vi "WILT Valve Test.vi"(0 "Water Valves Cluster":T8, 1 "Test Type":T7=enum."Full Valve Control", 2 "Operation Type":T11=enum."Operate As Stand-Alone EXE", 3 "Valve ON Time":dbl=100.0, 5 "Start Buttons Cluster":T9, 7 "Station Test State In":T5, 9 "Station Number":i32, 11 "Error In":errorcluster, 12 "Injection Times":T4, 13 "Day/Night Cycle":T10) -> (4 "Valve Actuation Complete":bool, 6 "Test Station Out":T5, 15 "Error Out":errorcluster)   [LabVIEW 2016]
uses:
  Type Definitions/WILT Water Valve Test Type.ctl
  Type Definitions/WILT Water Valve EXE Operation Type.ctl
  Type Definitions/WILT Water Valve Cluster.ctl
  Type Definitions/WILT Start Button Cluster.ctl
  Type Definitions/WILT Station Test State Cluster.ctl
  Type Definitions/WILT Dryer Test State.ctl
  Type Definitions/WILT Water Injection Control.ctl
  Type Definitions/WILT Day Night Cycle Enum.ctl
  Type Definitions/WILT Agilent Channel Definition.ctl
  Type Definitions/WILT Agilent Data Cluster.ctl
  <vilib>/Utility/error.llb/whitespace.ctl
  Drivers/Agilent 34972/Agilent 34970.lvlib
panel:
  out "Success":bool
  in  "Agilent Data In":T1
  out "Agilent Semaphore":T3[](array[typedef])
  in  "Agilent Switches":T2[](array[typedef])
  in  "Tab Control 2":enum32{"Water Valves", "Page 2"}(tab)
  out "Channel State?":string
  out "Agilent":T3
  in  "Tab Control":enum32{"Valve Setup", "Settings"}(tab)
  in  "Read Data":bool
  in  "Stop All Valves":bool
  in  "Shutdown All":bool
  in  "OK":bool
  in  "Number of ON/OFF Cycles":i32=1
  in  "Delay Before Valve ON":u32
  in  "Current Limit":dbl=1.0
  in  "Current Per Valve":dbl=0.42
  out "Label":string="Water Valve"
  out "Agilent Used":string="3"
  out "Channel Being Used":string="102"
  out "Agilent Data Out":T1
  out "Agilent Array":refnum<visa-resource-name>[](array[refnum])=["AGILENT2", "AGILENT2", "AGILENT2", "AGILENT2", "AGILENT2", "AGILENT2", "AGILENT2", "AGILENT2", "AGILENT2", "AGILENT2", "AGILENT2", "AGILENT2", "AGILENT2", "AGILENT2", "AGILENT2", "AGILENT2", "AGILENT2", "AGILENT2", "AGILENT2", "AGILENT2", "AGILENT3", "AGILENT3", "AGILENT3", "AGILENT3", "AGILENT3", "AGILENT3", "AGILENT3", "AGILENT3", "AGILENT3", "AGILENT3", "AGILENT3", "AGILENT3", "AGILENT5", "AGILENT5", "AGILENT5", "AGILENT5", "AGILENT5", "AGILENT5", "AGILENT5", "AGILENT5", "AGILENT5", "AGILENT5", "AGILENT5", "AGILENT5", "AGILENT5", "AGILENT5", "AGILENT5", "AGILENT5", "AGILENT5", "AGILENT5", "AGILENT5", "AGILENT5", "AGILENT5", "AGILENT5", "AGILENT5", "AGILENT5", "AGILENT5", "AGILENT5", "AGILENT5", "AGILENT5", "AGILENT5", "AGILENT5", "AGILENT5", "AGILENT5", "AGILENT5", "AGILENT5", "AGILENT5", "AGILENT5", "AGILENT7", "AGILENT7", "AGILENT7", "AGILENT7", "AGILENT7", "AGILENT7", "AGILENT7", "AGILENT7", "AGILENT7", "AGILENT7", "AGILENT7", "AGILENT7"]
  out "Agilent Channels":string[](array[string])=["301", "302", "303", "304", "305", "306", "307", "308", "309", "310", "311", "312", "313", "314", "315", "316", "317", "318", "319", "320", "101", "102", "103", "104", "105", "106", "107", "108", "109", "110", "111", "112", "101", "102", "103", "104", "105", "106", "107", "108", "109", "110", "111", "112", "113", "114", "115", "116", "117", "118", "119", "120", "201", "202", "203", "204", "301", "302", "303", "304", "305", "306", "307", "308", "309", "310", "311", "312", "101", "102", "103", "104", "105", "106", "107", "108", "109", "110", "111", "112"]
  out "Start Buttons":string[][](array[string])
  out "Water Valves":string[][](array[string])
  in  "Agilent Channel Assignment":path=path "C:/Work/Agilent Channel Assignment - Wilt.ini"
  out "Message":string
  # "100 ms is good for start switch"
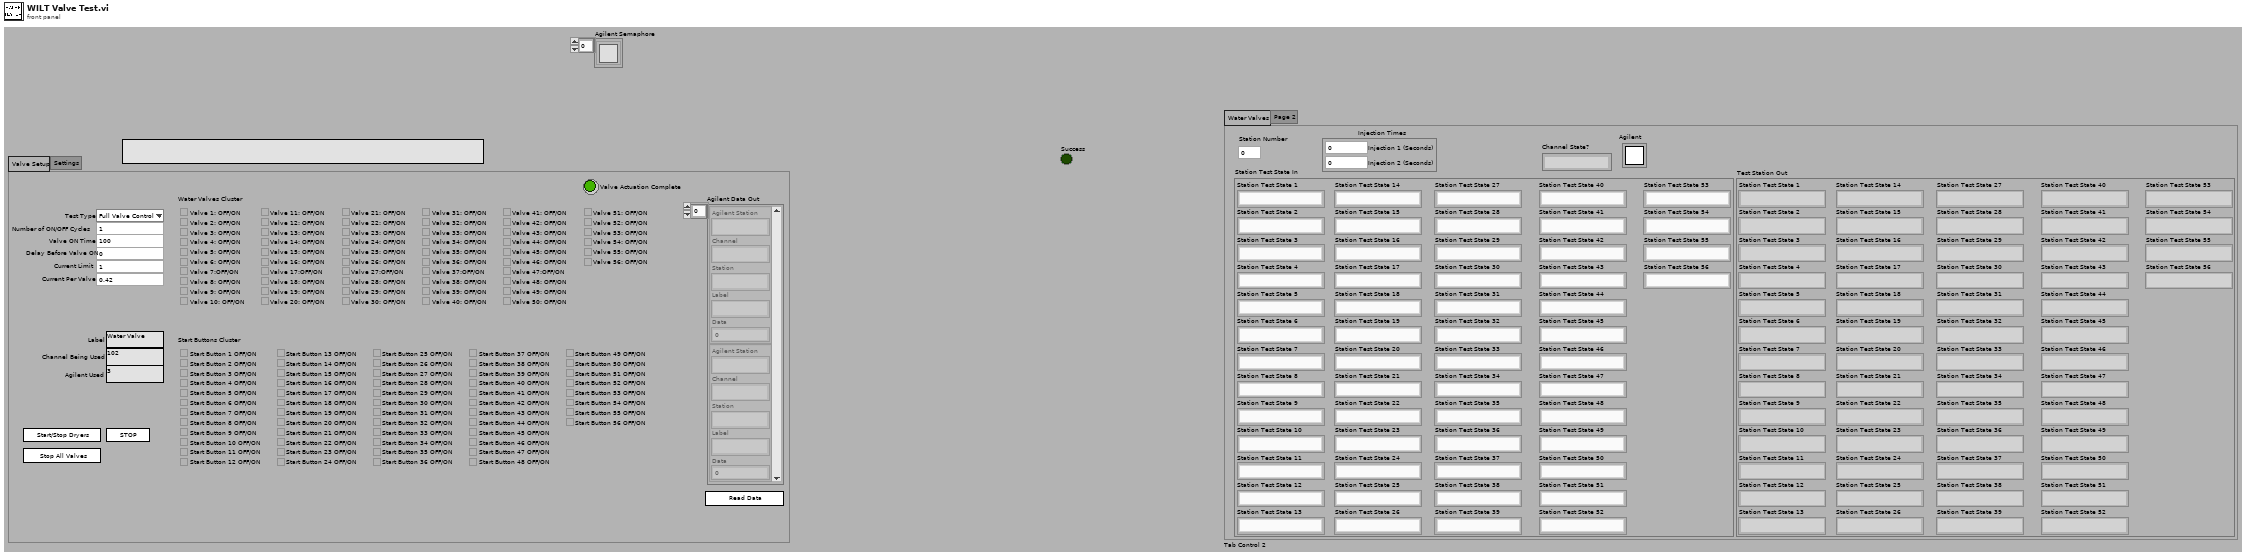
[diagram p1: front panel]
types:
  T1 = typedef "WILT Agilent Data Cluster.ctl" = T2[]
  T2 = typedef "WILT Agilent Channel Definition.ctl" = cluster{"Channel":string, "Station":string, "Label":string, "Agilent Station":string, "Data":dbl}
  T3 = typedef "Semaphore RefNum" = refnum<k1>
  T4 = typedef "WILT Water Injection Control.ctl" = cluster{"Injection 1 (Seconds)":dbl, "Injection 2 (Seconds)":dbl}
  T5 = typedef "WILT Station Test State Cluster.ctl" = cluster{"Station Test State 1":T6, "Station Test State 2":T6, "Station Test State 3":T6, "Station Test State 4":T6, "Station Test State 5":T6, "Station Test State 6":T6, "Station Test State 7":T6, "Station Test State 8":T6, "Station Test State 9":T6, "Station Test State 10":T6, "Station Test State 11":T6, "Station Test State 12":T6, "Station Test State 13":T6, "Station Test State 14":T6, "Station Test State 15":T6, "Station Test State 16":T6, "Station Test State 17":T6, "Station Test State 18":T6, "Station Test State 19":T6, "Station Test State 20":T6, "Station Test State 21":T6, "Station Test State 22":T6, "Station Test State 23":T6, "Station Test State 24":T6, "Station Test State 25":T6, "Station Test State 26":T6, "Station Test State 27":T6, "Station Test State 28":T6, "Station Test State 29":T6, "Station Test State 30":T6, "Station Test State 31":T6, "Station Test State 32":T6, "Station Test State 33":T6, "Station Test State 34":T6, "Station Test State 35":T6, "Station Test State 36":T6, "Station Test State 37":T6, "Station Test State 38":T6, "Station Test State 39":T6, "Station Test State 40":T6, "Station Test State 41":T6, "Station Test State 42":T6, "Station Test State 43":T6, "Station Test State 44":T6, "Station Test State 45":T6, "Station Test State 46":T6, "Station Test State 47":T6, "Station Test State 48":T6, "Station Test State 49":T6, "Station Test State 50":T6, "Station Test State 51":T6, "Station Test State 52":T6, "Station Test State 53":T6, "Station Test State 54":T6, "Station Test State 55":T6, "Station Test State 56":T6}
  T6 = typedef "WILT Dryer Test State.ctl" = enum16{"No Serial Number", "Waiting for Dryer To Start", "Drying Clothes", "Water Injection 1 (On)", "Water Injection 1 Timer", "Water Injection 1 (Off)", "Pause Dryer", "Sending Start Stop CMD", "Pause Dryer 2", "Sending Start Stop CMD 2", "Drying Clothes 2", "Water Injection 2 (On)", "Water Injection 2 Timer", "Water Injection 2 (Off)", "Drying Clothes 3", "Cooling Down", "Sending Start Stop CMD 3", "Increment Cycle"}
  T7 = typedef "WILT Water Valve Test Type.ctl" = enum16{"Cycle Valve Control", "Full Valve Control"}
  T8 = typedef "WILT Water Valve Cluster.ctl" = cluster{"Valve 1":bool, "Valve 2":bool, "Valve 3":bool, "Valve 4":bool, "Valve 5":bool, "Valve 6":bool, "Valve 7":bool, "Valve 8":bool, "Valve 9":bool, "Valve 10":bool, "Valve 11":bool, "Valve 12":bool, "Valve 13":bool, "Valve 14":bool, "Valve 15":bool, "Valve 16":bool, "Valve 17":bool, "Valve 18":bool, "Valve 19":bool, "Valve 20":bool, "Valve 21":bool, "Valve 22":bool, "Valve 23":bool, "Valve 24":bool, "Valve 25":bool, "Valve 26":bool, "Valve 27":bool, "Valve 28":bool, "Valve 29":bool, "Valve 30":bool, "Valve 31":bool, "Valve 32":bool, "Valve 33":bool, "Valve 34":bool, "Valve 35":bool, "Valve 36":bool, "Valve 37":bool, "Valve 38":bool, "Valve 39":bool, "Valve 40":bool, "Valve 41":bool, "Valve 42":bool, "Valve 43":bool, "Valve 44":bool, "Valve 45":bool, "Valve 46":bool, "Valve 47":bool, "Valve 48":bool, "Valve 49":bool, "Valve 50":bool, "Valve 51":bool, "Valve 52":bool, "Valve 53":bool, "Valve 54":bool, "Valve 55":bool, "Valve 56":bool}
  T9 = typedef "WILT Start Button Cluster.ctl" = cluster{"Start Button 21":bool, "Start Button 22":bool, "Start Button 23":bool, "Start Button 24":bool, "Start Button 25":bool, "Start Button 26":bool, "Start Button 27":bool, "Start Button 28":bool, "Start Button 29":bool, "Start Button 30":bool, "Start Button 31":bool, "Start Button 32":bool, "Start Button 33":bool, "Start Button 34":bool, "Start Button 35":bool, "Start Button 36":bool, "Start Button 37":bool, "Start Button 38":bool, "Start Button 39":bool, "Start Button 40":bool, "Start Button 41":bool, "Start Button 42":bool, "Start Button 43":bool, "Start Button 44":bool, "Start Button 12":bool, "Start Button 11":bool, "Start Button 10":bool, "Start Button 9":bool, "Start Button 8":bool, "Start Button 7":bool, "Start Button 6":bool, "Start Button 5":bool, "Start Button 4":bool, "Start Button 3":bool, "Start Button 2":bool, "Start Button 1":bool, "Start Button 20":bool, "Start Button 19":bool, "Start Button 18":bool, "Start Button 17":bool, "Start Button 16":bool, "Start Button 15":bool, "Start Button 14":bool, "Start Button 13":bool, "Start Button 45":bool, "Start Button 46":bool, "Start Button 47":bool, "Start Button 48":bool, "Start Button 49":bool, "Start Button 50":bool, "Start Button 51":bool, "Start Button 52":bool, "Start Button 53":bool, "Start Button 54":bool, "Start Button 55":bool, "Start Button 56":bool}
  T10 = typedef "WILT Day Night Cycle Enum.ctl" = enum16{"Day Cycle", "Night Cycle", "Day Cycle (No Water)"}
  T11 = typedef "WILT Water Valve EXE Operation Type.ctl" = enum16{"Operate As SubVI", "Operate As Stand-Alone EXE", "Shutdown All Dryers"}
  T12 = enum32{"invalid app kind", "Development System", "Run Time System", "Student Edition", "Embedded LabVIEW", "Evaluation", "Custom"}
  T13 = enum32{"Invalid", "Standard", "Closed", "Hidden", "Minimized", "Maximized"}
  T14 = cluster{"Core":cluster{"Current VI Reference":refnum<vi>, "Close Panel on Exit?":bool}, "Valve Array":bool[], "Water Valve Only":bool[], "Agilent":refnum<visa-resource-name>, "Channel":string, "Agilent Switches":T2[], "Agilent Array":refnum<visa-resource-name>[], "Agilent Channel Array":string[], "Start Buttons":string[][], "Water Valves":string[][], "Valve Act Complete":bool, "Water Valves Cluster":T8, "Start Buttons Cluster":T9, "Station Test State In":T5, "Agilent Data In":T1}
  T15 = cluster{"Current VI Reference":refnum<vi>, "Close Panel on Exit?":bool}
  T16 = typedef "whitespace.ctl" = u16
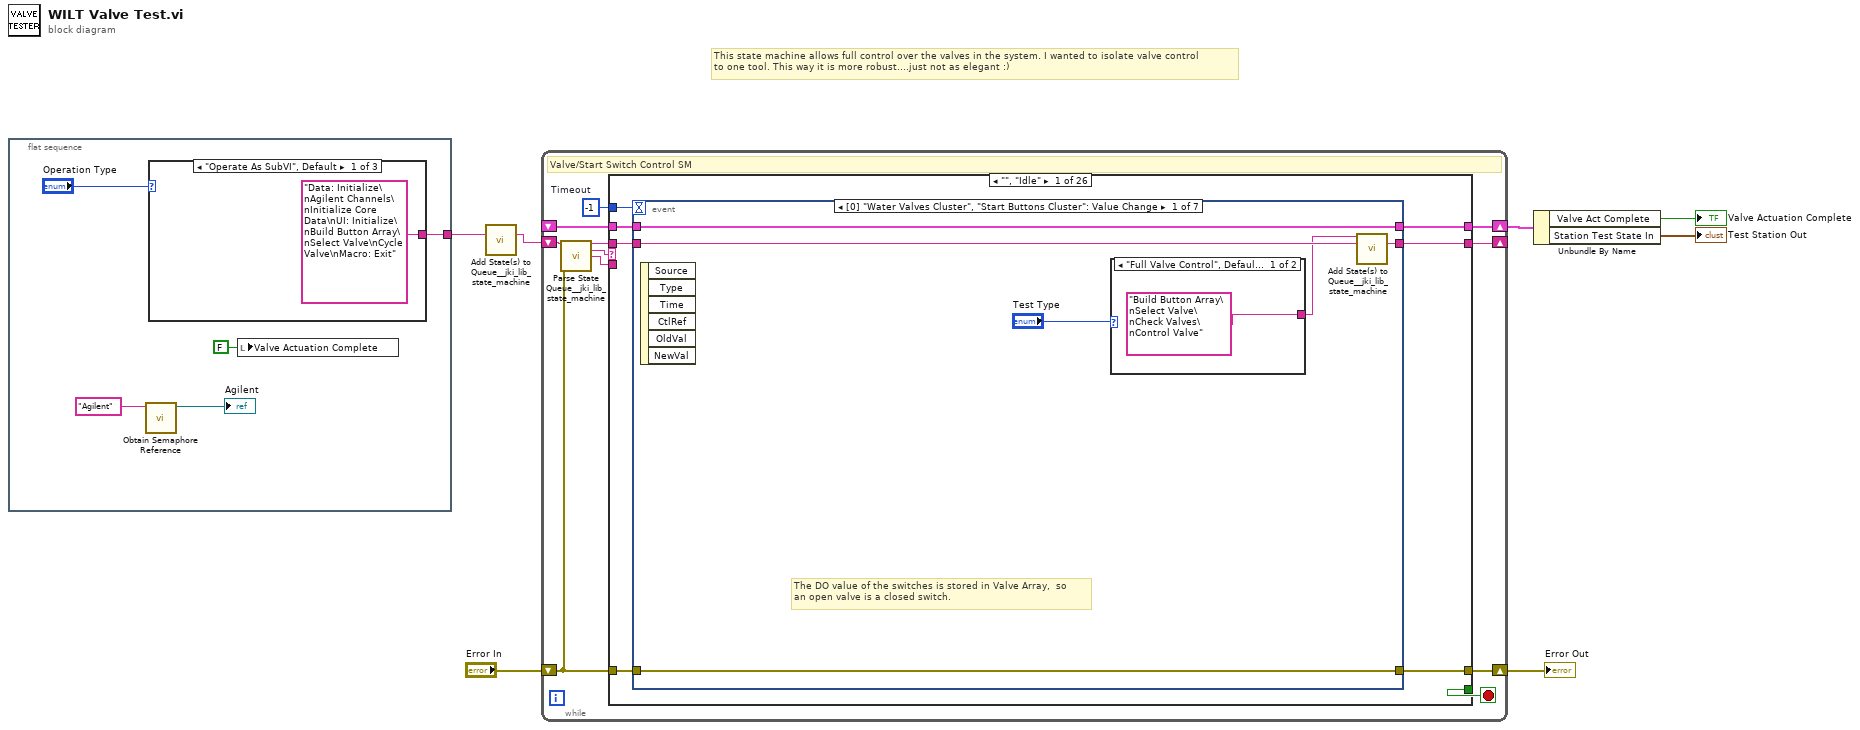
[diagram p0: block diagram]
diagram:
  # "This state machine allows full control over the valves in the system. I wanted to isolate valve control\nto one tool. This way it is more robust....just not as elegant :)"
  n1 = flat-sequence {
    tunnel: [w12] -> w6
    frame #0 {
      n2 = call <vilib>:"Obtain Semaphore Reference.vi"("name (unnamed)"="Agilent") -> ("semaphore"=→"Agilent":T3)  [unwired: 4 in, 2 out]
      n3 = case shown="\"Operate As SubVI\", Default" "Operation Type" {
        tunnel: ["Data: Initialize\nAgilent Channels\nInitialize Core Data\nUI: Initialize\nBuild Button Array\nSelect Valve\nCycle Valve\nMacro: Exit" ("State(s) in Front (\"\")") "Macro: Initialize" "Data: Initialize\nAgilent Channels\nInitialize Core Data\nUI: Initialize\nBuild Button Array\nSelect Valve\nShutdown All\nMacro: Exit" ("State(s) in Front (\"\")")] -> w12
        frame "Operate As SubVI", Default {
        }
        frame "Operate As Stand-Alone EXE" {
        }
        frame "Shutdown All Dryers" {
        }
      }
      n4 = local write "Valve Actuation Complete"(FALSE ("Valve Actuation Complete")) -> ()
    }
  }
  n5 = call <vilib>:"Add State(s) to Queue__jki_lib_state_machine.vi"("State(s) in (\"\")"=w6) -> ("States Out"=w7:string)  [unwired: 14 in]
  n6 = while "Valve/Start Switch Control SM" {
    shift-right: [w19] -> w3
    shift-left: _ -> [w18]
    shift-right: [w22] -> w5
    shift-left: "Error In" -> [w16]
    shift-right: [w21] -> _
    shift-left: w7 -> [w23]
    stop <- w20 stop-if-true
    w17 = -1  # Timeout
    # "Valve/Start Switch Control SM"
    n7 = call <vilib>:"Parse State Queue__jki_lib_state_machine.vi"("State Queue"=w23, "Error In (no error)"=w16) -> ("Remaining States"=w25:string, "Current State"=w26:string, "Arguments"=w24:string)  [unwired: 11 in]
    n8 = case shown="\"\", \"Idle\"" w26 {
      selector: w26 -> [_ _ w77 _ _ _ _ _ _ _ _ _ _ _ _ _ _ _ _ _ _ _ _ _ _ _]
      tunnel: w25 -> [w33 w76 w81 w99 w105 w110 w114 w133 w143 w155 w161 w165 w176 w1545 w1556 w1582 w1587 w1597 w1601 w1617 w1634 w1655 w1706 w1717 w1740 w1753]
      tunnel: w24 -> [_ _ _ _ _ _ _ _ _ _ _ _ _ w1540 w1550 _ _ _ _ _ _ _ _ _ _ _]
      tunnel: w18 -> [w31 w73 w79 w90 w102 w108 w111 _ w141 w147 w156 w162 w168 w1543 w1552 w1579 w1584 w1594 w1598 w1612 w1631 w1646 w1704 w1715 w1735 w1749]
      tunnel: [w30 w74 w83 w96 errorcluster {"status"=FALSE, "code"=0, "source"=""} ("error out") w107 w112 w130 w136 w150 w157 w163 w174 w1541 w1553 w1580 w1585 w1595 w1599 w1615 w1632 w1647 w1703 w1714 w1736 w1751] -> w22
      tunnel: w16 -> [w29 w74 w82 w96 w101 w107 w112 w130 w137 w152 w158 w163 w174 w1542 w1554 w1580 w1585 w1595 w1599 w1615 w1632 w1650 w1702 w1714 w1737 w1751]
      tunnel: [w32 w75 w80 w98 w104 w109 w113 w132 w142 w154 w160 w164 w175 w1544 w1555 w1581 w1586 w1596 w1600 w1616 w1633 w1654 w1705 w1716 w1739 w1752] -> w21
      tunnel: [_ _ _ _ _ TRUE _ _ _ _ _ _ _ _ _ _ _ _ _ _ _ _ _ _ _ _] -> w20
      tunnel: [w28 w73 w79 w97 w102 w108 w111 w131 w140 w146 w156 w162 w172 w1543 w1552 w1579 w1584 w1594 w1598 w1611 w1631 w1645 w1704 w1715 w1735 w1749] -> w19
      tunnel: w17 -> [w27 _ _ _ _ _ _ _ _ _ _ _ _ _ _ _ _ _ _ _ _ _ _ _ _ _]
      frame "", "Idle" {
        n9 = event shown="[0] \"Water Valves Cluster\", \"Start Buttons Cluster\": Value Change" {
          selector: _ -> [_ _ _ _ _ _ _]
          dyn-events: _ -> [_ _ _ _ _ _ _]
          timeout: w27 -> [_ _ _ _ _ _ _]
          tunnel: w33 -> [w39 w46 w51 w54 w58 w63 w72]
          tunnel: [w38 w45 w50 w53 w59 w64 w71] -> w32
          tunnel: w31 -> [w34 w43 w48 w55 w57 w65 w69]
          tunnel: [w37 w44 w49 w56 w61 w66 w70] -> w30
          tunnel: w29 -> [w37 w44 w49 w56 w61 w66 w70]
          tunnel: [w34 w43 w48 w55 w57 w65 w69] -> w28
          event Value Change {
            # "The DO value of the switches is stored in Valve Array,  so\nan open valve is a closed switch."
            n10 = event-data() -> ()  [unwired: 1 in, 6 out]
            n11 = case shown="\"Full Valve Control\", Default" "Test Type" {
              tunnel: ["Build Button Array\nSelect Valve\nCheck Valves\nControl Valve" ("State(s) in Front (\"\")") "Build Button Array\nSelect Valve\nCheck Valves\nCycle Valve" ("State(s) in Front (\"\")")] -> w36
              frame "Full Valve Control", Default {
              }
              frame "Cycle Valve Control" {
              }
            }
            n12 = call <vilib>:"Add State(s) to Queue__jki_lib_state_machine.vi"("State(s) in Front (\"\")"=w36, "State(s) in (\"\")"=w39) -> ("States Out"=w38:string)  [unwired: 13 in]
          }
          event Timeout {
            n13 = event-data() -> ()  [unwired: 1 in, 3 out]
            n14 = local write "Valve Actuation Complete"(FALSE ("Valve Actuation Complete")) -> ()
            n15 = call <vilib>:"Add State(s) to Queue__jki_lib_state_machine.vi"("State(s) in (\"\")"=w46) -> ("States Out"=w45:string)  [unwired: 14 in]
          }
          event "OK": Value Change {
            n16 = event-data() -> ()  [unwired: 1 in, 1 out]
            n17 = call <vilib>:"Add State(s) to Queue__jki_lib_state_machine.vi"("State(s) in Front (\"\")"="Macro: Exit", "State(s) in (\"\")"=w51) -> ("States Out"=w50:string)  [unwired: 13 in]
          }
          event "Shutdown All": Value Change {
            n18 = event-data() -> ()  [unwired: 1 in, 6 out]
            n19 = call <vilib>:"Add State(s) to Queue__jki_lib_state_machine.vi"("State(s) in Front (\"\")"="Stop All Valves\nShutdown All" ("State(s) in Front (\"\")"), "State(s) in (\"\")"=w54) -> ("States Out"=w53:string)  [unwired: 13 in]
          }
          event "Stop All Valves": Value Change {
            n20 = event-data() -> ()  [unwired: 1 in, 6 out]
            n21 = call <vilib>:"Add State(s) to Queue__jki_lib_state_machine.vi"("State(s) in Front (\"\")"="Stop All Valves" ("State(s) in Front (\"\")"), "State(s) in (\"\")"=w58) -> ("States Out"=w59:string)  [unwired: 13 in]
          }
          event "Read Data": Value Change {
            n22 = event-data() -> ()  [unwired: 1 in, 6 out]
            n23 = call <vilib>:"Add State(s) to Queue__jki_lib_state_machine.vi"("State(s) in Front (\"\")"="Read Agilents" ("name (unnamed)"), "State(s) in (\"\")"=w63) -> ("States Out"=w64:string)  [unwired: 13 in]
          }
          event Panel Close? {
            # "Discard the event because we'll close the front panel ourselves in Macro: Exit"
            # "Close Panel button (pressed) Event\n(this executes Macro: Exit to terminate the VI)"
            n24 = event-data() -> ()  [unwired: 1 in, 1 out]
            n25 = event-data("Discard?"=TRUE) -> ()  [unwired: 1 in, 1 out]
            n26 = call <vilib>:"Add State(s) to Queue__jki_lib_state_machine.vi"("State(s) in Front (\"\")"="Macro: Exit", "State(s) in (\"\")"=w72) -> ("States Out"=w71:string)  [unwired: 13 in]
          }
        }
      }
      frame "---------- Core ----------" {
        # "Do not put any code in this frame.\n(it is a separator no-op)"
        n27 = call <vilib>:"Add State(s) to Queue__jki_lib_state_machine.vi"("State(s) in (\"\")"=w76) -> ("States Out"=w75:string)  [unwired: 14 in]
      }
      frame Default {
        w86 = 42 items=["No error", "Argument error", "Memory is full", "Out of zone", "End of file", "File already open", "Generic file I/O error", "File not found", "File permission error", "Disk is full", "Duplicate path", "Too many files open", "System feature not enabled", "Resource file not found", "Cannot add resource", "Resource not found", "Image not found", "Image memory error", "Pen does not exist", "Config type invalid", "Config token not found", "Config parse error", "Config memory error", "Bad external code format", "Bad external code offset", "External code not present", "Null window", "Destroy window error", "Null menu", "Print aborted", "Bad print record", "Print driver error", "Windows error during printing", "Memory error during printing", "Print dialog error", "Generic print error", "Invalid device refnum", "Device not found", "Device parameter error", "Device unit error", "Cannot open device", "Device call aborted", "Generic error", "Cancelled by user", "Object ID too low", "Object ID too high", "Object not in heap", "Unknown heap", "Unknown object (invalid DefProc)", "Unknown object (DefProc not in table)", "Message out of range", "Invalid (null) method", "Unknown message", "Manager call not supported", "Bad address", "Network operation in progress", "Network operation timed out", "Connection is busy", "Network attribute not supported", "Network error", "Address in use", "System out of memory", "Connection aborted", "Connection refused", "Not connected", "Already connected", "Connection closed", "Initialization error (interapplication manager)", "Bad occurrence", "Wait on unbound occurrence handler", "Occurrence queue overflow", "Datalog type conflict", "Unused", "Unrecognized type (interapplication manager)", "Memory corrupt", "Failed to make temporary DLL", "Old CIN version", "Drag socket not found", "Failed to load drop-object", "Failed to register OLE object", "Failed to release OLE object", "Format specifier type mismatch", "Unknown format specifier", "Too few format specifiers", "Too many format specifiers", "Scan failed", "Newer CIN version", "Error converting to variant", "Runtime menu error", "Password tampered", "Variant attribute not found", "Incompatible variant data type", "Event data is not available", "Event Store is not present", "Occurrence is not found", "Event Queue is not created", "Event info is not available", "Refnum passed is NULL", "Error retrieving Class GUID", "Error retrieving CoClass GUID", "Error retrieving TypeLib GUID.", "Bad built application magic bytes.", "Specific driver is different from the specific driver associated with the Logical Name.", "There is no session opened to the class driver.", "Max Error", "MAX - Error with config objects", "MAX - Error loading configuration", "MAX - Group not supported"]
        # "Current State"
        # "Do not delete, rename, or modify this frame.\n(this is used to capture unhandled states and typos)"
        # "Handle mistyped state name (developer tool)"
        n28 = Format Into String(format string="Software Exception: Unhandled State \"%s\"." ("message"), error in=w82, w77) -> (resulting string=w85:string, error out=w84:errorcluster)  [unwired: 1 in]
        n29 = call <vilib>:"Error Cluster From Error Code.vi"("show call chain? (False)"=TRUE, "error in (no error)"=w84, "error message (\"\")"=w85, "error code (0)"=w86) -> ("error out"=w83:errorcluster)  [unwired: 5 in]
        n30 = call <vilib>:"Add State(s) to Queue__jki_lib_state_machine.vi"("State(s) in (\"\")"=w81) -> ("States Out"=w80:string)  [unwired: 14 in]
      }
      frame "Initialize Core Data" {
        # "Do not delete, rename, or modify this frame.\n(this is used to determine panel behavior on exit)"
        # "originally closed?"
        # "exe?"
        # "If panel starts closed or is an EXE, then close it when we exit"
        n31 = property class="VI"() -> ("Front Panel.Open"=w95:bool)  [unwired: 2 in, 2 out]
        n32 = property class="App"() -> ("App.Kind"=w94:T12)  [unwired: 2 in, 2 out]
        n33 = control-ref of="Current VI Reference"() -> (w88:refnum<vi>)
        n34 = Not(x=w95) -> (.not. x?=w92:bool)
        n35 = Equal?(x=w94, y=T12."Run Time System" ("Application:Kind")) -> (x = y?=w91:bool)
        n36 = Or(x=w92, y=w91) -> (x .or. y?=w89:bool)
        n37 = Bundle By Name(cluster=w90, "Core.Current VI Reference"=w88, "Core.Close Panel on Exit?"=w89) -> (w97:T14)
        n38 = call <vilib>:"Add State(s) to Queue__jki_lib_state_machine.vi"("State(s) in (\"\")"=w99) -> ("States Out"=w98:string)  [unwired: 14 in]
      }
      frame "Error Handler" {
        # "Unhandled Error -- Display it"
        # "Handle any errors here.\nYou can also output any states to clean-up after errors occur"
        # "Clear error"
        n39 = call <vilib>:"General Error Handler.vi"("error in (no error)"=w101) -> ()  [unwired: 10 in, 5 out]
        n40 = call <vilib>:"Add State(s) to Queue__jki_lib_state_machine.vi"("State(s) in Front (\"\")"="/* Post Error States", "State(s) in (\"\")"=w105) -> ("States Out"=w104:string)  [unwired: 13 in]
      }
      frame "Exit" {
        # "Do not put any code in this frame.\n(No errors that occur here will be handled.)"
        n41 = call <vilib>:"Add State(s) to Queue__jki_lib_state_machine.vi"("State(s) in (\"\")"=w110) -> ("States Out"=w109:string)  [unwired: 14 in]
      }
      frame "---------- Data ----------" {
        # "Do not put any code in this frame.\n(It is a separator no-op. You can make a copy of this frame to create a new Data frame)"
        n42 = call <vilib>:"Add State(s) to Queue__jki_lib_state_machine.vi"("State(s) in (\"\")"=w114) -> ("States Out"=w113:string)  [unwired: 14 in]
      }
      frame "Data: Initialize" {
        w121 = bool[] [FALSE, FALSE, FALSE, FALSE, FALSE, FALSE, FALSE, FALSE, FALSE, FALSE]  # Water Valve Only
        w126 = "1"  # Channel
        w127 = refnum<visa-resource-name> "AGILENT1"  # Agilent
        w128 = bool[] [FALSE, FALSE, FALSE, FALSE, FALSE, FALSE, FALSE, FALSE, FALSE, FALSE]  # Valve Array
        w129 = T15 {"Current VI Reference"=refnum, "Close Panel on Exit?"=FALSE}  # Core
        n43 = Bundle("Core"=w129, "Valve Array"=w128, "Water Valve Only"=w121, "Agilent"=w127, "Channel"=w126, "Agilent Switches"="Agilent Switches", "Agilent Array"=refnum<visa-resource-name>[] [], "Agilent Channel Array"=string[] [], "Start Buttons"=string[][] [], "Water Valves"=string[][] [], "Valve Act Complete"=FALSE, "Water Valves Cluster"="Water Valves Cluster", "Start Buttons Cluster"="Start Buttons Cluster", "Station Test State In"="Station Test State In", "Agilent Data In"="Agilent Data In") -> (w131:T14)  [unwired: 1 in]
        n44 = call <vilib>:"Add State(s) to Queue__jki_lib_state_machine.vi"("State(s) in (\"\")"=w133) -> ("States Out"=w132:string)  [unwired: 14 in]
      }
      frame "Agilent Channels" {
        n45 = disable-structure shown="Disabled" {
          frame Disabled {
            n46 = local read "Agilent"() -> ()  [unwired: 1 out]
          }
          frame Enabled {
          }
        }
        n47 = call "WILT Agilent Setup.vi"("Custom Agilent List"=TRUE, "Agilent Channel Assignment"="Agilent Channel Assignment", "error in (no error)"=w137, "Agilent Refs"=refnum<visa-resource-name>[] ["AGILENT1", "AGILENT2", "AGILENT3", "AGILENT4", "AGILENT5", "AGILENT6", "AGILENT7"]) -> ("error out"=w136:errorcluster, "Agilent Switches"=w139:T2[])  [unwired: 5 in, 1 out]
        n48 = Bundle By Name(cluster=w141, "Agilent Switches"=w139) -> (w140:T14)
        n49 = call <vilib>:"Add State(s) to Queue__jki_lib_state_machine.vi"("State(s) in (\"\")"=w143) -> ("States Out"=w142:string)  [unwired: 14 in]
      }
      frame "Build Button Array" {
        n50 = Unbundle By Name(w147) -> ("Agilent Switches"=w149:T2[])
        n51 = call "WILT Build Array of Start Buttons and Water Valves.vi"("Error In"=w152, "Agilent Valve and Switch Locations"=w149, "Label Search"="Start Button" ("y")) -> ("Error Out"=w151:errorcluster, "Array of Values"=w144:string[][])  [unwired: 7 in]
        "Start Buttons" <- w144
        n52 = call "WILT Build Array of Start Buttons and Water Valves.vi"("Error In"=w151, "Agilent Valve and Switch Locations"=w149, "Label Search"="Water Valve" ("y")) -> ("Error Out"=w150:errorcluster, "Array of Values"=w145:string[][])  [unwired: 7 in]
        "Water Valves" <- w145
        n53 = Bundle By Name(cluster=w147, "Start Buttons"=w144, "Water Valves"=w145) -> (w146:T14)
        n54 = call <vilib>:"Add State(s) to Queue__jki_lib_state_machine.vi"("State(s) in (\"\")"=w155) -> ("States Out"=w154:string)  [unwired: 14 in]
      }
      frame "Data: Cleanup" {
        # "Cleanup any data and references, here.\n(this is called automatically, by the Macro: Exit)"
        n55 = Unbundle By Name(w156) -> ("Core.Current VI Reference"=w159:refnum<vi>)
        n56 = Close Reference(reference=w159, error in (no error)=w158) -> (error out=w157:errorcluster)
        n57 = call <vilib>:"Add State(s) to Queue__jki_lib_state_machine.vi"("State(s) in (\"\")"=w161) -> ("States Out"=w160:string)  [unwired: 14 in]
      }
      frame "---------- UI ----------" {
        # "Do not put any code in this frame.\n(It is a separator no-op. You can make a copy of this frame to create a new UI frame)"
        n58 = call <vilib>:"Add State(s) to Queue__jki_lib_state_machine.vi"("State(s) in (\"\")"=w165) -> ("States Out"=w164:string)  [unwired: 14 in]
      }
      frame "UI: Initialize" {
        # "Initialize everything if running as a EXE\nDont initialize becasue I will feed an \narray and dont want to clear for SubVI"
        n59 = local read "Operation Type"() -> (w169:T11)
        n60 = Unbundle By Name(w168) -> ("Station Test State In"=w166:T5, "Agilent Switches"=w173:T2[])
        n61 = case shown="\"Operate As SubVI\", Default" w169 {
          tunnel: w168 -> [w182 w1533]
          tunnel: [w181 w1532] -> w167
          tunnel: w166 -> [w179 _]
          frame "Operate As SubVI", Default {
            n62 = case shown="22" "Station Number" {
              tunnel: w179 -> [_ w189 w213 w237 w261 w285 w309 w333 w357 w381 w405 w429 w453 w477 w501 w525 w549 w573 w597 w621 w645 w669 w693 w717 w741 w765 w789 w813 w837 w861 w885 w909 w933 w957 w981 w1005 w1029 w1053 w1077 w1101 w1125 w1149 w1173 w1197 w1221 w1245 w1269 w1293 w1317 w1341 w1365 w1389 w1413 w1437 w1461 w1485 w1509]
              tunnel: [WILT_Dryer_Test_State."No Serial Number" ("Station Test State 56") w187 w210 w236 w260 w284 w306 w332 w354 w380 w404 w426 w452 w476 w500 w524 w548 w572 w596 w620 w642 w668 w692 w716 w740 w764 w788 w812 w836 w860 w884 w908 w932 w956 w980 w1004 w1028 w1052 w1076 w1100 w1124 w1148 w1172 w1196 w1220 w1244 w1268 w1292 w1316 w1340 w1364 w1388 w1412 w1436 w1460 w1484 w1508] -> _
              tunnel: [T8 {"Valve 1"=FALSE, "Valve 2"=FALSE, "Valve 3"=FALSE, "Valve 4"=FALSE, "Valve 5"=FALSE, "Valve 6"=FALSE, "Valve 7"=FALSE, "Valve 8"=FALSE, "Valve 9"=FALSE, "Valve 10"=FALSE, "Valve 11"=FALSE, "Valve 12"=FALSE, "Valve 13"=FALSE, "Valve 14"=FALSE, "Valve 15"=FALSE, "Valve 16"=FALSE, "Valve 17"=FALSE, "Valve 18"=FALSE, "Valve 19"=FALSE, "Valve 20"=FALSE, "Valve 21"=FALSE, "Valve 22"=FALSE, "Valve 23"=FALSE, "Valve 24"=FALSE, "Valve 25"=FALSE, "Valve 26"=FALSE, "Valve 27"=FALSE, "Valve 28"=FALSE, "Valve 29"=FALSE, "Valve 30"=FALSE, "Valve 31"=FALSE, "Valve 32"=FALSE, "Valve 33"=FALSE, "Valve 34"=FALSE, "Valve 35"=FALSE, "Valve 36"=FALSE, "Valve 37"=FALSE, "Valve 38"=FALSE, "Valve 39"=FALSE, "Valve 40"=FALSE, "Valve 41"=FALSE, "Valve 42"=FALSE, "Valve 43"=FALSE, "Valve 44"=FALSE, "Valve 45"=FALSE, "Valve 46"=FALSE, "Valve 47"=FALSE, "Valve 48"=FALSE, "Valve 49"=FALSE, "Valve 50"=FALSE, "Valve 51"=FALSE, "Valve 52"=FALSE, "Valve 53"=FALSE, "Valve 54"=FALSE, "Valve 55"=FALSE, "Valve 56"=FALSE} ("Water Valves Cluster") w188 w212 w235 w259 w283 w308 w331 w356 w379 w403 w428 w451 w475 w499 w523 w547 w571 w595 w619 w644 w667 w691 w715 w739 w763 w787 w811 w835 w859 w883 w907 w931 w955 w979 w1003 w1027 w1051 w1075 w1099 w1123 w1147 w1171 w1195 w1219 w1243 w1267 w1291 w1315 w1339 w1363 w1387 w1411 w1435 w1459 w1483 w1507] -> w178
              tunnel: [T9 {"Start Button 21"=FALSE, "Start Button 22"=FALSE, "Start Button 23"=FALSE, "Start Button 24"=FALSE, "Start Button 25"=FALSE, "Start Button 26"=FALSE, "Start Button 27"=FALSE, "Start Button 28"=FALSE, "Start Button 29"=FALSE, "Start Button 30"=FALSE, "Start Button 31"=FALSE, "Start Button 32"=FALSE, "Start Button 33"=FALSE, "Start Button 34"=FALSE, "Start Button 35"=FALSE, "Start Button 36"=FALSE, "Start Button 37"=FALSE, "Start Button 38"=FALSE, "Start Button 39"=FALSE, "Start Button 40"=FALSE, "Start Button 41"=FALSE, "Start Button 42"=FALSE, "Start Button 43"=FALSE, "Start Button 44"=FALSE, "Start Button 12"=FALSE, "Start Button 11"=FALSE, "Start Button 10"=FALSE, "Start Button 9"=FALSE, "Start Button 8"=FALSE, "Start Button 7"=FALSE, "Start Button 6"=FALSE, "Start Button 5"=FALSE, "Start Button 4"=FALSE, "Start Button 3"=FALSE, "Start Button 2"=FALSE, "Start Button 1"=FALSE, "Start Button 20"=FALSE, "Start Button 19"=FALSE, "Start Button 18"=FALSE, "Start Button 17"=FALSE, "Start Button 16"=FALSE, "Start Button 15"=FALSE, "Start Button 14"=FALSE, "Start Button 13"=FALSE, "Start Button 45"=FALSE, "Start Button 46"=FALSE, "Start Button 47"=FALSE, "Start Button 48"=FALSE, "Start Button 49"=FALSE, "Start Button 50"=FALSE, "Start Button 51"=FALSE, "Start Button 52"=FALSE, "Start Button 53"=FALSE, "Start Button 54"=FALSE, "Start Button 55"=FALSE, "Start Button 56"=FALSE} ("Start Buttons Cluster") w186 w211 w234 w258 w282 w307 w330 w355 w378 w402 w427 w450 w474 w498 w522 w546 w570 w594 w618 w643 w666 w690 w714 w738 w762 w786 w810 w834 w858 w882 w906 w930 w954 w978 w1002 w1026 w1050 w1074 w1098 w1122 w1146 w1170 w1194 w1218 w1242 w1266 w1290 w1314 w1338 w1362 w1386 w1410 w1434 w1458 w1482 w1506] -> w177
              frame 0, Default {
                # "This is not a station.\nDo nothing"
              }
              frame 1 {
                n63 = Unbundle By Name(w189) -> ("Station Test State 1"=w187:T6)
                n64 = case shown="\"Sending Start Stop CMD 3\"" w187 {
                  tunnel: [w191 w195 T8 {"Valve 1"=FALSE, "Valve 2"=FALSE, "Valve 3"=FALSE, "Valve 4"=FALSE, "Valve 5"=FALSE, "Valve 6"=FALSE, "Valve 7"=FALSE, "Valve 8"=FALSE, "Valve 9"=FALSE, "Valve 10"=FALSE, "Valve 11"=FALSE, "Valve 12"=FALSE, "Valve 13"=FALSE, "Valve 14"=FALSE, "Valve 15"=FALSE, "Valve 16"=FALSE, "Valve 17"=FALSE, "Valve 18"=FALSE, "Valve 19"=FALSE, "Valve 20"=FALSE, "Valve 21"=FALSE, "Valve 22"=FALSE, "Valve 23"=FALSE, "Valve 24"=FALSE, "Valve 25"=FALSE, "Valve 26"=FALSE, "Valve 27"=FALSE, "Valve 28"=FALSE, "Valve 29"=FALSE, "Valve 30"=FALSE, "Valve 31"=FALSE, "Valve 32"=FALSE, "Valve 33"=FALSE, "Valve 34"=FALSE, "Valve 35"=FALSE, "Valve 36"=FALSE, "Valve 37"=FALSE, "Valve 38"=FALSE, "Valve 39"=FALSE, "Valve 40"=FALSE, "Valve 41"=FALSE, "Valve 42"=FALSE, "Valve 43"=FALSE, "Valve 44"=FALSE, "Valve 45"=FALSE, "Valve 46"=FALSE, "Valve 47"=FALSE, "Valve 48"=FALSE, "Valve 49"=FALSE, "Valve 50"=FALSE, "Valve 51"=FALSE, "Valve 52"=FALSE, "Valve 53"=FALSE, "Valve 54"=FALSE, "Valve 55"=FALSE, "Valve 56"=FALSE} ("Water Valves Cluster") T8 {"Valve 1"=FALSE, "Valve 2"=FALSE, "Valve 3"=FALSE, "Valve 4"=FALSE, "Valve 5"=FALSE, "Valve 6"=FALSE, "Valve 7"=FALSE, "Valve 8"=FALSE, "Valve 9"=FALSE, "Valve 10"=FALSE, "Valve 11"=FALSE, "Valve 12"=FALSE, "Valve 13"=FALSE, "Valve 14"=FALSE, "Valve 15"=FALSE, "Valve 16"=FALSE, "Valve 17"=FALSE, "Valve 18"=FALSE, "Valve 19"=FALSE, "Valve 20"=FALSE, "Valve 21"=FALSE, "Valve 22"=FALSE, "Valve 23"=FALSE, "Valve 24"=FALSE, "Valve 25"=FALSE, "Valve 26"=FALSE, "Valve 27"=FALSE, "Valve 28"=FALSE, "Valve 29"=FALSE, "Valve 30"=FALSE, "Valve 31"=FALSE, "Valve 32"=FALSE, "Valve 33"=FALSE, "Valve 34"=FALSE, "Valve 35"=FALSE, "Valve 36"=FALSE, "Valve 37"=FALSE, "Valve 38"=FALSE, "Valve 39"=FALSE, "Valve 40"=FALSE, "Valve 41"=FALSE, "Valve 42"=FALSE, "Valve 43"=FALSE, "Valve 44"=FALSE, "Valve 45"=FALSE, "Valve 46"=FALSE, "Valve 47"=FALSE, "Valve 48"=FALSE, "Valve 49"=FALSE, "Valve 50"=FALSE, "Valve 51"=FALSE, "Valve 52"=FALSE, "Valve 53"=FALSE, "Valve 54"=FALSE, "Valve 55"=FALSE, "Valve 56"=FALSE} ("Water Valves Cluster") T8 {"Valve 1"=FALSE, "Valve 2"=FALSE, "Valve 3"=FALSE, "Valve 4"=FALSE, "Valve 5"=FALSE, "Valve 6"=FALSE, "Valve 7"=FALSE, "Valve 8"=FALSE, "Valve 9"=FALSE, "Valve 10"=FALSE, "Valve 11"=FALSE, "Valve 12"=FALSE, "Valve 13"=FALSE, "Valve 14"=FALSE, "Valve 15"=FALSE, "Valve 16"=FALSE, "Valve 17"=FALSE, "Valve 18"=FALSE, "Valve 19"=FALSE, "Valve 20"=FALSE, "Valve 21"=FALSE, "Valve 22"=FALSE, "Valve 23"=FALSE, "Valve 24"=FALSE, "Valve 25"=FALSE, "Valve 26"=FALSE, "Valve 27"=FALSE, "Valve 28"=FALSE, "Valve 29"=FALSE, "Valve 30"=FALSE, "Valve 31"=FALSE, "Valve 32"=FALSE, "Valve 33"=FALSE, "Valve 34"=FALSE, "Valve 35"=FALSE, "Valve 36"=FALSE, "Valve 37"=FALSE, "Valve 38"=FALSE, "Valve 39"=FALSE, "Valve 40"=FALSE, "Valve 41"=FALSE, "Valve 42"=FALSE, "Valve 43"=FALSE, "Valve 44"=FALSE, "Valve 45"=FALSE, "Valve 46"=FALSE, "Valve 47"=FALSE, "Valve 48"=FALSE, "Valve 49"=FALSE, "Valve 50"=FALSE, "Valve 51"=FALSE, "Valve 52"=FALSE, "Valve 53"=FALSE, "Valve 54"=FALSE, "Valve 55"=FALSE, "Valve 56"=FALSE} ("Water Valves Cluster")] -> w188
                  tunnel: [T9 {"Start Button 21"=FALSE, "Start Button 22"=FALSE, "Start Button 23"=FALSE, "Start Button 24"=FALSE, "Start Button 25"=FALSE, "Start Button 26"=FALSE, "Start Button 27"=FALSE, "Start Button 28"=FALSE, "Start Button 29"=FALSE, "Start Button 30"=FALSE, "Start Button 31"=FALSE, "Start Button 32"=FALSE, "Start Button 33"=FALSE, "Start Button 34"=FALSE, "Start Button 35"=FALSE, "Start Button 36"=FALSE, "Start Button 37"=FALSE, "Start Button 38"=FALSE, "Start Button 39"=FALSE, "Start Button 40"=FALSE, "Start Button 41"=FALSE, "Start Button 42"=FALSE, "Start Button 43"=FALSE, "Start Button 44"=FALSE, "Start Button 12"=FALSE, "Start Button 11"=FALSE, "Start Button 10"=FALSE, "Start Button 9"=FALSE, "Start Button 8"=FALSE, "Start Button 7"=FALSE, "Start Button 6"=FALSE, "Start Button 5"=FALSE, "Start Button 4"=FALSE, "Start Button 3"=FALSE, "Start Button 2"=FALSE, "Start Button 1"=FALSE, "Start Button 20"=FALSE, "Start Button 19"=FALSE, "Start Button 18"=FALSE, "Start Button 17"=FALSE, "Start Button 16"=FALSE, "Start Button 15"=FALSE, "Start Button 14"=FALSE, "Start Button 13"=FALSE, "Start Button 45"=FALSE, "Start Button 46"=FALSE, "Start Button 47"=FALSE, "Start Button 48"=FALSE, "Start Button 49"=FALSE, "Start Button 50"=FALSE, "Start Button 51"=FALSE, "Start Button 52"=FALSE, "Start Button 53"=FALSE, "Start Button 54"=FALSE, "Start Button 55"=FALSE, "Start Button 56"=FALSE} ("Start Buttons Cluster") T9 {"Start Button 21"=FALSE, "Start Button 22"=FALSE, "Start Button 23"=FALSE, "Start Button 24"=FALSE, "Start Button 25"=FALSE, "Start Button 26"=FALSE, "Start Button 27"=FALSE, "Start Button 28"=FALSE, "Start Button 29"=FALSE, "Start Button 30"=FALSE, "Start Button 31"=FALSE, "Start Button 32"=FALSE, "Start Button 33"=FALSE, "Start Button 34"=FALSE, "Start Button 35"=FALSE, "Start Button 36"=FALSE, "Start Button 37"=FALSE, "Start Button 38"=FALSE, "Start Button 39"=FALSE, "Start Button 40"=FALSE, "Start Button 41"=FALSE, "Start Button 42"=FALSE, "Start Button 43"=FALSE, "Start Button 44"=FALSE, "Start Button 12"=FALSE, "Start Button 11"=FALSE, "Start Button 10"=FALSE, "Start Button 9"=FALSE, "Start Button 8"=FALSE, "Start Button 7"=FALSE, "Start Button 6"=FALSE, "Start Button 5"=FALSE, "Start Button 4"=FALSE, "Start Button 3"=FALSE, "Start Button 2"=FALSE, "Start Button 1"=FALSE, "Start Button 20"=FALSE, "Start Button 19"=FALSE, "Start Button 18"=FALSE, "Start Button 17"=FALSE, "Start Button 16"=FALSE, "Start Button 15"=FALSE, "Start Button 14"=FALSE, "Start Button 13"=FALSE, "Start Button 45"=FALSE, "Start Button 46"=FALSE, "Start Button 47"=FALSE, "Start Button 48"=FALSE, "Start Button 49"=FALSE, "Start Button 50"=FALSE, "Start Button 51"=FALSE, "Start Button 52"=FALSE, "Start Button 53"=FALSE, "Start Button 54"=FALSE, "Start Button 55"=FALSE, "Start Button 56"=FALSE} ("Start Buttons Cluster") w199 w202 w206] -> w186
                  frame "Water Injection 1 (On)", Default {
                    n65 = Bundle By Name(cluster=T8 {"Valve 1"=FALSE, "Valve 2"=FALSE, "Valve 3"=FALSE, "Valve 4"=FALSE, "Valve 5"=FALSE, "Valve 6"=FALSE, "Valve 7"=FALSE, "Valve 8"=FALSE, "Valve 9"=FALSE, "Valve 10"=FALSE, "Valve 11"=FALSE, "Valve 12"=FALSE, "Valve 13"=FALSE, "Valve 14"=FALSE, "Valve 15"=FALSE, "Valve 16"=FALSE, "Valve 17"=FALSE, "Valve 18"=FALSE, "Valve 19"=FALSE, "Valve 20"=FALSE, "Valve 21"=FALSE, "Valve 22"=FALSE, "Valve 23"=FALSE, "Valve 24"=FALSE, "Valve 25"=FALSE, "Valve 26"=FALSE, "Valve 27"=FALSE, "Valve 28"=FALSE, "Valve 29"=FALSE, "Valve 30"=FALSE, "Valve 31"=FALSE, "Valve 32"=FALSE, "Valve 33"=FALSE, "Valve 34"=FALSE, "Valve 35"=FALSE, "Valve 36"=FALSE, "Valve 37"=FALSE, "Valve 38"=FALSE, "Valve 39"=FALSE, "Valve 40"=FALSE, "Valve 41"=FALSE, "Valve 42"=FALSE, "Valve 43"=FALSE, "Valve 44"=FALSE, "Valve 45"=FALSE, "Valve 46"=FALSE, "Valve 47"=FALSE, "Valve 48"=FALSE, "Valve 49"=FALSE, "Valve 50"=FALSE, "Valve 51"=FALSE, "Valve 52"=FALSE, "Valve 53"=FALSE, "Valve 54"=FALSE, "Valve 55"=FALSE, "Valve 56"=FALSE} ("Water Valves Cluster"), "Valve 1"=TRUE) -> (w191:T8)
                  }
                  frame "Drying Clothes 2" {
                    n66 = Bundle By Name(cluster=T8 {"Valve 1"=FALSE, "Valve 2"=FALSE, "Valve 3"=FALSE, "Valve 4"=FALSE, "Valve 5"=FALSE, "Valve 6"=FALSE, "Valve 7"=FALSE, "Valve 8"=FALSE, "Valve 9"=FALSE, "Valve 10"=FALSE, "Valve 11"=FALSE, "Valve 12"=FALSE, "Valve 13"=FALSE, "Valve 14"=FALSE, "Valve 15"=FALSE, "Valve 16"=FALSE, "Valve 17"=FALSE, "Valve 18"=FALSE, "Valve 19"=FALSE, "Valve 20"=FALSE, "Valve 21"=FALSE, "Valve 22"=FALSE, "Valve 23"=FALSE, "Valve 24"=FALSE, "Valve 25"=FALSE, "Valve 26"=FALSE, "Valve 27"=FALSE, "Valve 28"=FALSE, "Valve 29"=FALSE, "Valve 30"=FALSE, "Valve 31"=FALSE, "Valve 32"=FALSE, "Valve 33"=FALSE, "Valve 34"=FALSE, "Valve 35"=FALSE, "Valve 36"=FALSE, "Valve 37"=FALSE, "Valve 38"=FALSE, "Valve 39"=FALSE, "Valve 40"=FALSE, "Valve 41"=FALSE, "Valve 42"=FALSE, "Valve 43"=FALSE, "Valve 44"=FALSE, "Valve 45"=FALSE, "Valve 46"=FALSE, "Valve 47"=FALSE, "Valve 48"=FALSE, "Valve 49"=FALSE, "Valve 50"=FALSE, "Valve 51"=FALSE, "Valve 52"=FALSE, "Valve 53"=FALSE, "Valve 54"=FALSE, "Valve 55"=FALSE, "Valve 56"=FALSE} ("Water Valves Cluster"), "Valve 1"=TRUE) -> (w195:T8)
                  }
                  frame "Sending Start Stop CMD" {
                    n67 = Bundle By Name(cluster=T9 {"Start Button 21"=FALSE, "Start Button 22"=FALSE, "Start Button 23"=FALSE, "Start Button 24"=FALSE, "Start Button 25"=FALSE, "Start Button 26"=FALSE, "Start Button 27"=FALSE, "Start Button 28"=FALSE, "Start Button 29"=FALSE, "Start Button 30"=FALSE, "Start Button 31"=FALSE, "Start Button 32"=FALSE, "Start Button 33"=FALSE, "Start Button 34"=FALSE, "Start Button 35"=FALSE, "Start Button 36"=FALSE, "Start Button 37"=FALSE, "Start Button 38"=FALSE, "Start Button 39"=FALSE, "Start Button 40"=FALSE, "Start Button 41"=FALSE, "Start Button 42"=FALSE, "Start Button 43"=FALSE, "Start Button 44"=FALSE, "Start Button 12"=FALSE, "Start Button 11"=FALSE, "Start Button 10"=FALSE, "Start Button 9"=FALSE, "Start Button 8"=FALSE, "Start Button 7"=FALSE, "Start Button 6"=FALSE, "Start Button 5"=FALSE, "Start Button 4"=FALSE, "Start Button 3"=FALSE, "Start Button 2"=FALSE, "Start Button 1"=FALSE, "Start Button 20"=FALSE, "Start Button 19"=FALSE, "Start Button 18"=FALSE, "Start Button 17"=FALSE, "Start Button 16"=FALSE, "Start Button 15"=FALSE, "Start Button 14"=FALSE, "Start Button 13"=FALSE, "Start Button 45"=FALSE, "Start Button 46"=FALSE, "Start Button 47"=FALSE, "Start Button 48"=FALSE, "Start Button 49"=FALSE, "Start Button 50"=FALSE, "Start Button 51"=FALSE, "Start Button 52"=FALSE, "Start Button 53"=FALSE, "Start Button 54"=FALSE, "Start Button 55"=FALSE, "Start Button 56"=FALSE} ("Start Buttons Cluster"), "Start Button 1"=TRUE ("Start Button 21")) -> (w199:T9)
                  }
                  frame "Sending Start Stop CMD 2" {
